vi "Q -- range -- gate  - OR.vi"(3 "new state":T1=enum."above", 4 "gate":T1=enum."above") -> (0 "new state out":T1)   [LabVIEW 2010]
uses:
  comparison control.ctl
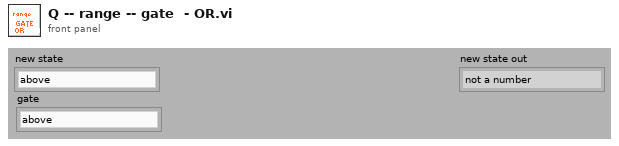
[diagram p1: front panel]
types:
  T1 = typedef "comparison control.ctl" = enum16{"not a number", "above", "in range", "below"}
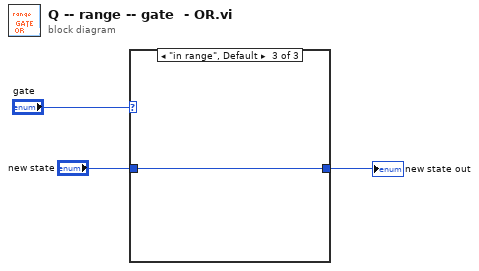
[diagram p0: block diagram]
diagram:
  n1 = case shown="\"in range\", Default" "gate" {
    selector: "gate" -> [w4 w5 _]
    tunnel: [w4 w5 w6] -> w3
    tunnel: "new state" -> [_ _ w6]
    frame "above" {
    }
    frame "below" {
    }
    frame "in range", Default {
    }
  }
  "new state out" <- w3
